vi "Get Biometry Average Data General.vi"(8 "error in (no error)":errorcluster caption="错误输入（无错误）", 10 "condition":string, 11 "connection reference":T1) -> (0 "error out":errorcluster caption="错误输出", 2 "Data Output":string[][](array[string]))   [LabVIEW 2015, in "Utility VIs.lvlib"]
doc: "该模板用于创建子VI。"
uses:
  Utility VIs.lvlib
  <vilib>/addons/database/Connection.llb/Conn ObjectReference.ctl
  Database Processing/Database Processing.lvlib
  <vilib>/addons/database/NI_Database_API.lvlib
panel:
  # "Busy"
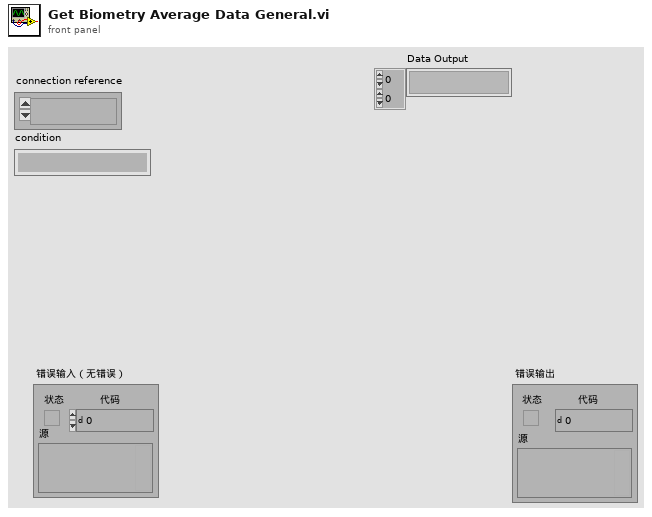
[diagram p1: front panel]
types:
  T1 = typedef "NI_Database_API.lvlib/Conn ObjectReference.ctl" = refnum<k1>
  T2 = typedef "Database Processing.lvlib/Biometry Average Attribute.ctl" = cluster{"Parameter_ID":i64, "Measure_No":i64, "L_Or_R":string}
  T3 = typedef "Database Processing.lvlib/Biometry Average Parameter.ctl" = cluster{"Parameter_ID":i64, "Central_Corneal_Thickness":sgl, "Anterior_Chamber_Depth":sgl, "Len_Thickness":sgl, "Retinal_Thickness":sgl, "Axis_Length":sgl, "Pupil_Diameter":sgl, "PCX":sgl, "PCY":sgl, "White_To_White":sgl, "ICX":sgl, "ICY":sgl, "Keratometric_flat":sgl, "Keratometric_steep":sgl, "Keratometric_Axis(flat)":sgl, "Keratometric_Axis(steep)":sgl, "Keratometric_AST":sgl}
  T4 = typedef "Database Processing.lvlib/Biometry Average State.ctl" = cluster{"Parameter_ID":i64, "Central_Corneal_Thickness_State":string, "Anterior_Chamber_Depth_State":string, "Len_Thickness_State":string, "Retinal_Thickness_State":string, "Axis_Length_State":string, "Pupil_Diameter_State":string, "White_To_White_State":string, "Keratometric_flat_State":string, "Keratometric_steep_State":string}
  T5 = typedef "Database Processing.lvlib/Biometry Average Standard Deviation.ctl" = cluster{"Parameter_ID":i64, "Central_Corneal_Thickness":sgl, "Anterior_Chamber_Depth":sgl, "Len_Thickness":sgl, "Retinal_Thickness":sgl, "Axis_Length":sgl, "Pupil_Diameter":sgl, "PCX":sgl, "PCY":sgl, "White_To_White":sgl, "ICX":sgl, "ICY":sgl, "Keratometric_flat":sgl, "Keratometric_steep":sgl, "Keratometric_Axis(flat)":sgl, "Keratometric_Axis(steep)":sgl, "Keratometric_AST":sgl}
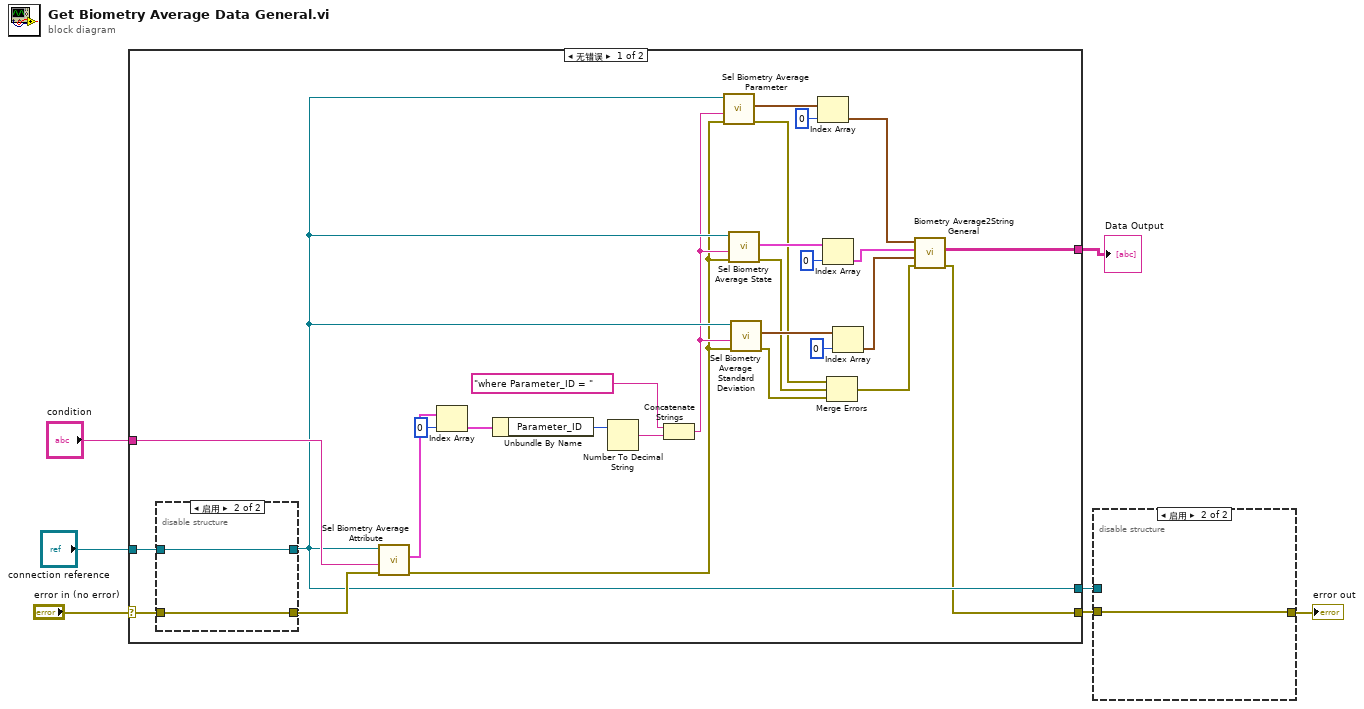
[diagram p0: block diagram]
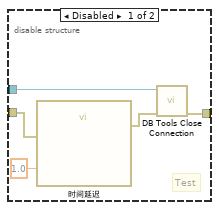
[diagram p2: hidden frame]
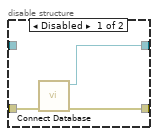
[diagram p3: hidden frame]
diagram:
  n1 = case shown="无错误" "error in (no error)" {
    selector: "error in (no error)" -> [w35 w42]
    tunnel: [w9 w42] -> w4
    tunnel: "connection reference" -> [w34 w41]
    tunnel: "condition" -> [w32 _]
    tunnel: [w21 w41] -> w2
    tunnel: [w8 _] -> w1
    frame No Error {
      n2 = disable-structure shown="启用" {
        disable-tunnel: w35 -> [w38 w39]
        disable-tunnel: w34 -> [_ w40]
        disable-tunnel: [w37 w40] -> w21
        disable-tunnel: [w36 w39] -> w33
        frame Disabled {
          n3 = call "Connect Database.vi"("error in (no error)"=w38) -> ("error out"=w36:errorcluster, "connection reference"=w37:T1)  [unwired: 9 in]
        }
        frame Enabled {
        }
      }
      n4 = call "Sel Biometry Average Attribute.vi"("error in (no error)"=w33, "condition"=w32, "connection reference"=w21) -> ("error out"=w19:errorcluster, "Biometry Average Attribute"=w31:T2[])  [unwired: 7 in]
      n5 = Index Array(array=w31, index=0 ("索引")) -> (element=w29:T2)
      n6 = Unbundle By Name(w29) -> ("Parameter_ID"=w27:i64)
      n7 = Number To Decimal String(number=w27) -> (decimal integer string=w28:string)  [unwired: 1 in]
      n8 = Concatenate Strings("where Parameter_ID = " ("字符串"), w28) -> (w20:string)
      n9 = call "Sel Biometry Average Parameter.vi"("error in (no error)"=w19, "condition"=w20, "connection reference"=w21) -> ("error out"=w13:errorcluster, "Biometry Average Parameter"=w24:T3[])  [unwired: 7 in]
      n10 = call "Sel Biometry Average State.vi"("error in (no error)"=w19, "condition"=w20, "connection reference"=w21) -> ("error out"=w12:errorcluster, "Biometry Average State"=w22:T4[])  [unwired: 7 in]
      n11 = call "Sel Biometry Average Standard Deviation.vi"("error in (no error)"=w19, "condition"=w20, "connection reference"=w21) -> ("error out"=w11:errorcluster, "Biometry_Average_Standard_Deviation"=w17:T5[])  [unwired: 7 in]
      n12 = Index Array(array=w24, index=0 ("索引")) -> (element=w16:T3)
      n13 = Index Array(array=w22, index=0 ("索引")) -> (element=w15:T4)
      n14 = Merge Errors(w13, w12, w11) -> (w10:errorcluster)
      n15 = Index Array(array=w17, index=0 ("索引")) -> (element=w14:T5)
      n16 = call "Biometry Average2String General.vi"("error in (no error)"=w10, "Biometry Average Standard Deviation"=w14, "Biometry Average State"=w15, "Biometry Average Parameter"=w16) -> ("error out"=w9:errorcluster, "Data Output"=w8:string[][])  [unwired: 6 in]
    }
    frame Error {
    }
  }
  "Data Output" <- w1
  n17 = disable-structure shown="启用" {
    disable-tunnel: w4 -> [w45 w48]
    disable-tunnel: [w47 w48] -> w3
    disable-tunnel: w2 -> [w46 _]
    frame Disabled {
      # "Test"
      n18 = call "时间延迟"("error in (no error)"=w45, "Delay Time (s)"=1.0) -> ("error out"=w44:errorcluster)  [unwired: 9 in]
      n19 = call <vilib>:"DB Tools Close Connection.vi"("error in (no error)"=w44, "connection reference"=w46) -> ("error out"=w47:errorcluster)  [unwired: 5 in]
    }
    frame Enabled {
    }
  }
  "error out" <- w3
